vi "Set Capacity Limits.vi"(6 "parseError? T:Yes":bool=TRUE, 8 "error in (no error)":errorcluster, 9 "Maximum cooling capacity(-100%)":i8 min=-100 max=0, 10 "Maximum heating capacity(100%)":u8=100 max=100, 11 "VISA resource name":refnum<visa-resource-name>) -> (0 "error out":errorcluster, 3 "VISA resource name out":refnum<visa-resource-name>)   [LabVIEW 2018, in "JULABO DeviceDriver.lvlib"]
doc: "This VI adjusts the maximum allowed heating and cooling capacity in percent. 100 % corresponds to the technical specification of the equipment.\nAdjustable range: \nHeating capacity: <B>0 ... 100 %</B>\nCooling capacity: <B>-100 ... 0 % </B>\n\nValues outside the allowed range are coerced to fit the valid range and no error occurs.\n\nNote:\nThe maximum cooling capacity is only adjustable for models with <B>proportional cooling control</B>."
uses:
  JULABO DeviceDriver.lvlib
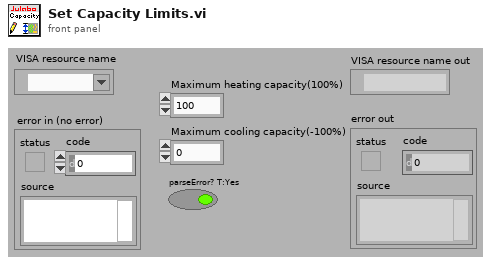
[diagram p1: front panel]
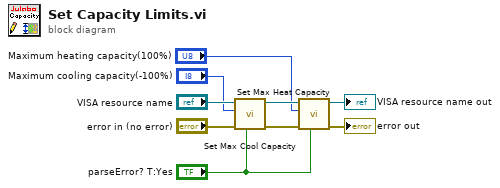
[diagram p0: block diagram]
diagram:
  n1 = call "Set Max Cool Capacity.vi"("parseError? T:Yes"="parseError? T:Yes", "error in (no error)"="error in (no error)", "Maximum cooling capacity(-100%)"="Maximum cooling capacity(-100%)", "VISA resource name"="VISA resource name") -> ("error out"=w6:errorcluster, "VISA resource name out"=w7:refnum<visa-resource-name>)  [unwired: 6 in]
  n2 = call "Set Max Heat Capacity.vi"("parseError? T:Yes"="parseError? T:Yes", "error in (no error)"=w6, "Maximum heating capacity(100%)"="Maximum heating capacity(100%)", "VISA resource name"=w7) -> ("error out"=→"error out":errorcluster, "VISA resource name out"=→"VISA resource name out":refnum<visa-resource-name>)  [unwired: 6 in]
